vi "5668 Scan with External LO Fetch Data.vi"(8 "error in (no error)":errorcluster, 10 "timeout (10 sec)":dbl=10.0, 11 "Instrument Handles in":T1={"Resource Name RFSA"="RFSA", "Resource Name RFSG LO Generation"="RFSG"}) -> (0 "error out":errorcluster, 2 "Data":waveform(cdb)[](array[waveform]), 3 "Instrument Handles out":T1={"Resource Name RFSA"="RFSA", "Resource Name RFSG LO Generation"="RFSG"})   [LabVIEW 2017]
uses:
  Instrument Handles.ctl
  <instrlib>/niRFSA/niRFSA.llb/niRFSA Fetch IQ (1D Complex WDT NRec 1Chan).vi
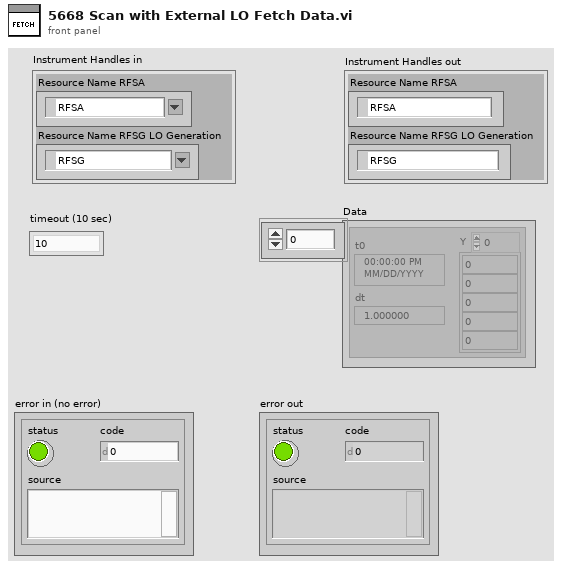
[diagram p1: front panel]
types:
  T1 = typedef "Instrument Handles.ctl" = cluster{"Resource Name RFSA":refnum<k15>, "Resource Name RFSG LO Generation":refnum<k15>}
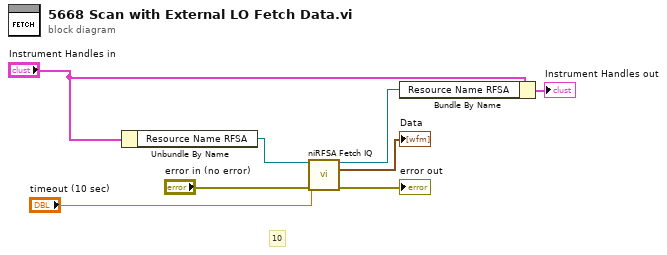
[diagram p0: block diagram]
diagram:
  # "10"
  n1 = Unbundle By Name("Instrument Handles in") -> ("Resource Name RFSA"=w5:refnum<k15>)
  n2 = call-poly <instrlib>:"niRFSA Fetch IQ.vi"("instrument handle"=w5, "timeout (10 sec)"="timeout (10 sec)", "error in"="error in (no error)") -> ("instrument handle out"=w4:refnum<k15>, "data"=→"Data":waveform(cdb)[], "error out"=→"error out":errorcluster)  [unwired: 10 in]
  n3 = Bundle By Name(cluster="Instrument Handles in", "Resource Name RFSA"=w4) -> (→"Instrument Handles out":T1)
